vi "PDC_RAWFileLoad.vi"(0 "FileName":string, 1 "ImageBuffInfo":T1, 2 "RawBitDepth":u32, 3 "error in (no error)":errorcluster) -> (5 "Data(16Bit)":u16[](array[numeric]), 6 "Data(8Bit)":u8[](array[numeric]), 7 "ReturnValue":u32, 8 "ErrorCode":u32, 10 "error out":errorcluster)   [LabVIEW 8.6]
doc: "This VI acquires the image data from RAW/RAWW file."
uses:
  PDCLIB.dll
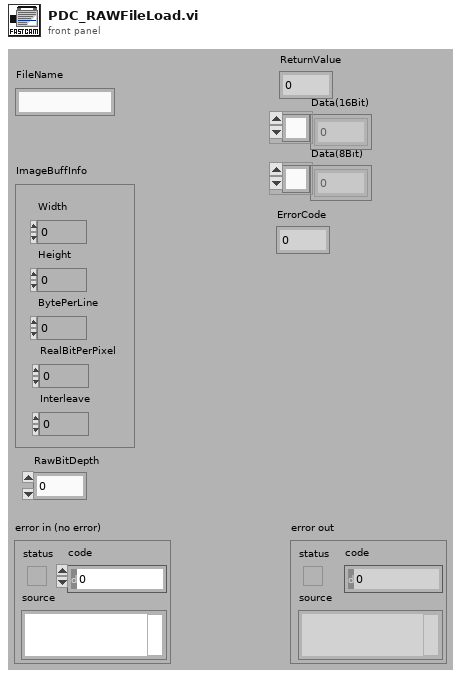
[diagram p1: front panel]
types:
  T1 = cluster{"Width":i32, "Height":i32, "BytePerLine":i32, "RealBitPerPixel":u16, "Interleave":i32}
  T2 = cluster{"Width":i32, "Height":i32, "BytePerLine":i32, "RealBitPerPixel":u16, u16, "Interleave":i32}
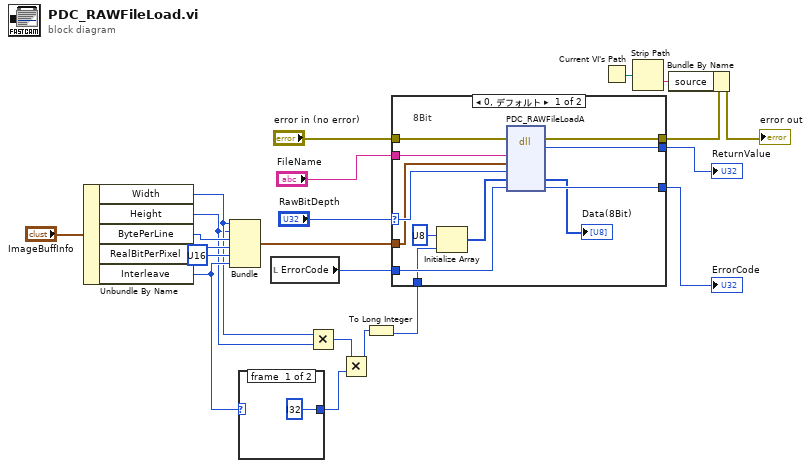
[diagram p0: block diagram]
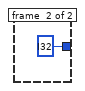
[diagram p2: hidden frame]
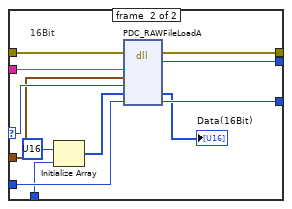
[diagram p3: hidden frame]
diagram:
  n1 = Unbundle By Name("ImageBuffInfo") -> ("Width"=w2:i32, "Height"=w1:i32, "BytePerLine"=w7:i32, "RealBitPerPixel"=w6:u16, "Interleave"=w3:i32)
  n2 = Bundle("Width"=w2, "Height"=w1, "BytePerLine"=w7, "RealBitPerPixel"=w6, u16 ?, "Interleave"=w3) -> (w4:T2)  [unwired: 1 in]
  n3 = case shown="1, 2" w3 {
    tunnel: [i32 ? ("y") i32 ? ("y")] -> w17
    frame #0 {
    }
    frame #1 {
    }
  }
  n4 = local read "ErrorCode"() -> (w20:u32)
  n5 = Multiply(x=w2, y=w1) -> (x*y=w18:i32)
  n6 = Multiply(x=w18, y=w17) -> (x*y=w16:i32)
  n7 = To Long Integer(number=w16) -> (32bit integer=w11:i32)
  n8 = case shown="0, デフォルト" "RawBitDepth" {
    selector: "RawBitDepth" -> [w26 w39]
    tunnel: [w36 w48] -> w22
    tunnel: [w35 w47] -> w13
    tunnel: "error in (no error)" -> [w34 w46]
    tunnel: w20 -> [w33 w45]
    tunnel: [w32 w44] -> w19
    tunnel: w11 -> [w29 w41]
    tunnel: "FileName" -> [w27 w38]
    tunnel: w4 -> [w25 w37]
    frame #0 {
      # "8Bit"
      n9 = Initialize Array(u8 ? ("要素"), w29) -> (w28:u8[])
      n10 = dll-call lib="PDCLIB.dll" fn="PDC_RAWFileLoadA"(error in=w34, "nFileName"=w27, "pInfo"=w25, "nRawBitDepth"=w26, "pBuff"=w28, "pErrorCode"=w33) -> (error out=w35:errorcluster, "return type"=w36:u32, "pBuff"=→"Data(8Bit)":u8[], "pErrorCode"=w32:u32)  [unwired: 5 in, 1 out]
    }
    frame #1 {
      # "16Bit"
      n11 = Initialize Array(u16 ? ("要素"), w41) -> (w40:u16[])
      n12 = dll-call lib="PDCLIB.dll" fn="PDC_RAWFileLoadA"(error in=w46, "nFileName"=w38, "pInfo"=w37, "nRawBitDepth"=w39, "pData"=w40, "pErrorCode"=w45) -> (error out=w47:errorcluster, "return type"=w48:u32, "pData"=→"Data(16Bit)":u16[], "pErrorCode"=w44:u32)  [unwired: 5 in, 1 out]
    }
  }
  "ReturnValue" <- w22
  "ErrorCode" <- w19
  n13 = Current VI's Path() -> (path=w14:path)
  n14 = Strip Path(path=w14) -> (name=w15:string)  [unwired: 1 out]
  n15 = Bundle By Name(cluster=w13, "source"=w15) -> (→"error out":errorcluster)
